vi "set_duration.vi"(8 "error in (no error)":errorcluster, 10 "duration":dbl[unit], 11 "DAQ_MG090622Camera in":refnum<class "DAQ_MG090622Camera.lvclass">) -> (0 "error out":errorcluster, 3 "DAQ_MG090622Camera out":refnum<class "DAQ_MG090622Camera.lvclass">)   [LabVIEW 2010, in "DAQ_MG090622Camera.lvclass"]
uses:
  DAQ_MG090622Camera.lvclass
  DAQ_MG090622Camera.lvclass/DAQ_MG090622Camera.ctl
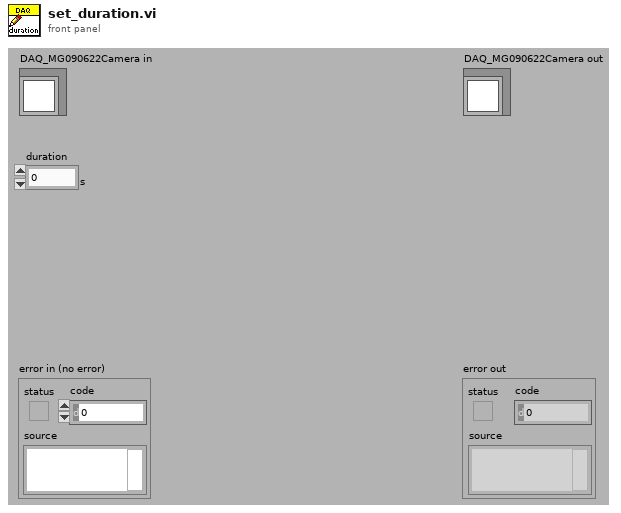
[diagram p1: front panel]
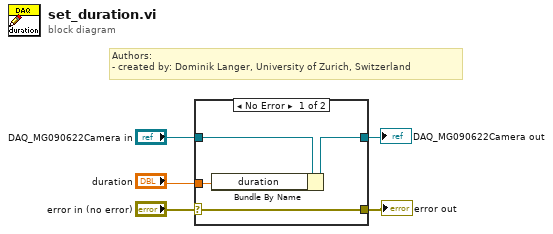
[diagram p0: block diagram]
diagram:
  # "Authors: \n- created by: Dominik Langer, University of Zurich, Switzerland"
  n1 = case shown="No Error" "error in (no error)" {
    selector: "error in (no error)" -> [w9 w10]
    tunnel: [w9 w10] -> w4
    tunnel: [w7 w11] -> w2
    tunnel: "DAQ_MG090622Camera in" -> [w8 w11]
    tunnel: "duration" -> [w6 _]
    frame No Error {
      n2 = Bundle By Name(cluster=w8, "duration"=w6) -> (w7:refnum<class "DAQ_MG090622Camera.lvclass">)
    }
    frame Error {
    }
  }
  "error out" <- w4
  "DAQ_MG090622Camera out" <- w2
